vi "test_Checksum U8 - Add Protection.vi"(8 "error in (no error)":errorcluster) -> (0 "error out":errorcluster)   [LabVIEW 2023, in "Instrument Addon Protections Unit Tests.lvclass"]
uses:
  Instrument Addon Protections Unit Tests.lvclass
  <vilib>/addons/_JKI Toolkits/VI Tester/TestCase.llb/TestCase.lvclass
  Checksum U8/Checksum U8.lvclass
panel:
  out "Checksum U8 out":refnum<class "Checksum U8.lvclass">
  in  "Checksum U8 in":refnum<class "Checksum U8.lvclass">
  out "TestCase out":refnum<class "Instrument Addon Protections Unit Tests.lvclass">
  in  "TestCase in":refnum<class "Instrument Addon Protections Unit Tests.lvclass">
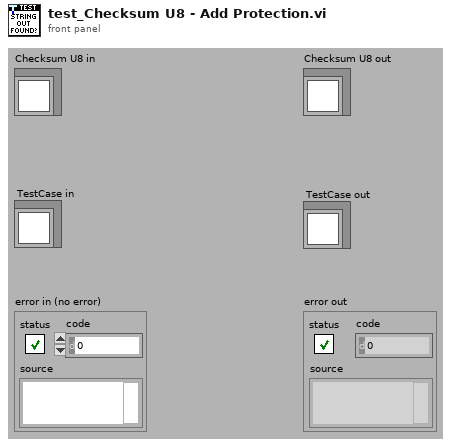
[diagram p1: front panel]
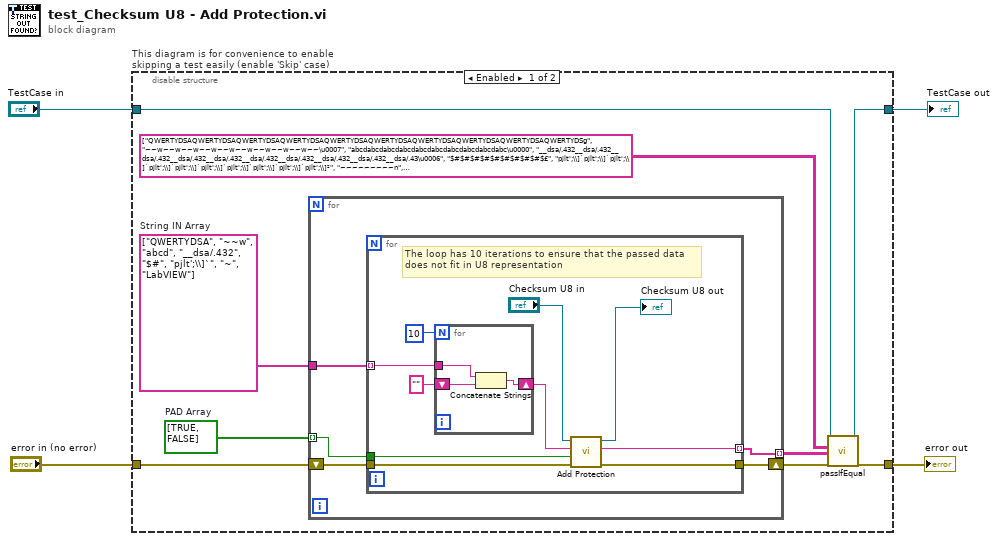
[diagram p0: block diagram]
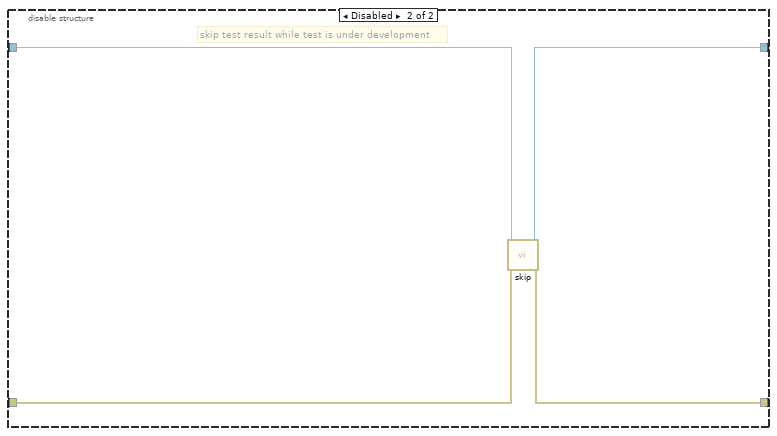
[diagram p2: hidden frame]
diagram:
  n1 = disable-structure "This diagram is for convenience to enable skipping a test easily (enable 'Skip' case)" shown="Enabled" {
    disable-tunnel: "TestCase in" -> [w11 w35]
    disable-tunnel: [w12 w33] -> w1
    disable-tunnel: [w13 w34] -> w3
    disable-tunnel: "error in (no error)" -> [w10 w32]
    frame Enabled {
      w6 = string[] ["QWERTYDSA", "~~w", "abcd", "__dsa/.432", "$#", "pjlt';\\]`", "~", "LabVIEW"]  # String IN Array
      w7 = bool[] [TRUE, FALSE]  # PAD Array
      n2 = for {
        tunnel: [w17] -> w9 mode=indexing
        shift-right: [w16] -> w8
        shift-left: w10 -> [w18]
        tunnel: w7 -> [w15] mode=indexing
        tunnel: w6 -> [w14]
        n3 = for {
          tunnel: w14 -> [w26] mode=indexing
          tunnel: w18 -> [w25]
          tunnel: [w24] -> w16
          tunnel: [w23] -> w17 mode=indexing
          tunnel: w15 -> [w22]
          # "The loop has 10 iterations to ensure that the passed data\ndoes not fit in U8 representation"
          n4 = for {
            N: 10 -> [_]
            shift-right: [w31] -> w21
            shift-left: "" -> [w30]
            tunnel: w26 -> [w29]
            n5 = Concatenate Strings(w29, w30) -> (w31:string)
          }
          n6 = call-dynamic "Add Protection.vi"("error in (no error)"=w25, "Pad"=w22, "String in"=w21, "Checksum U8 in"="Checksum U8 in") -> ("error out"=w24:errorcluster, "String out"=w23:string, "Checksum U8 out"=→"Checksum U8 out":refnum<class "Checksum U8.lvclass">)  [unwired: 5 in]
        }
      }
      n7 = call-dynamic "passIfEqual.vi"("error in (no error)"=w8, "y"=w9, "x"=string[][] [["QWERTYDSAQWERTYDSAQWERTYDSAQWERTYDSAQWERTYDSAQWERTYDSAQWERTYDSAQWERTYDSAQWERTYDSAQWERTYDSg", "~~w~~w~~w~~w~~w~~w~~w~~w~~w~~\u0007", "abcdabcdabcdabcdabcdabcdabcdabcdabcdabc\u0000", "__dsa/.432__dsa/.432__dsa/.432__dsa/.432__dsa/.432__dsa/.432__dsa/.432__dsa/.432__dsa/.432__dsa/.43\u0006", "$#$#$#$#$#$#$#$#$#$£", "pjlt';\\]`pjlt';\\]`pjlt';\\]`pjlt';\\]`pjlt';\\]`pjlt';\\]`pjlt';\\]`pjlt';\\]`pjlt';\\]`pjlt';\\]²", "~~~~~~~~~n", "LabVIEWLabVIEWLabVIEWLabVIEWLabVIEWLabVIEWLabVIEWLabVIEWLabVIEWLabVIE"], ["QWERTYDSAQWERTYDSAQWERTYDSAQWERTYDSAQWERTYDSAQWERTYDSAQWERTYDSAQWERTYDSAQWERTYDSAQWERTYDSA¨", "~~w~~w~~w~~w~~w~~w~~w~~w~~w~~w~", "abcdabcdabcdabcdabcdabcdabcdabcdabcdabcdd", "__dsa/.432__dsa/.432__dsa/.432__dsa/.432__dsa/.432__dsa/.432__dsa/.432__dsa/.432__dsa/.432__dsa/.4328", "$#$#$#$#$#$#$#$#$#$#Æ", "pjlt';\\]`pjlt';\\]`pjlt';\\]`pjlt';\\]`pjlt';\\]`pjlt';\\]`pjlt';\\]`pjlt';\\]`pjlt';\\]`pjlt';\\]`\u0012", "~~~~~~~~~~ì", "LabVIEWLabVIEWLabVIEWLabVIEWLabVIEWLabVIEWLabVIEWLabVIEWLabVIEWLabVIEWä"]] ("Array"), "TestCase in"=w11) -> ("error out"=w13:errorcluster, "TestCase out"=w12:refnum<class "Instrument Addon Protections Unit Tests.lvclass">)  [unwired: 6 in]
    }
    frame Disabled {
      # "skip test result while test is under development"
      n8 = call <vilib>:"skip.vi"("error in (no error)"=w32, "TestCase in"=w35) -> ("error out"=w34:errorcluster, "TestCase out"=w33:refnum<class "Instrument Addon Protections Unit Tests.lvclass">)  [unwired: 8 in]
    }
  }
  "error out" <- w3
  "TestCase out" <- w1
